vi "Conversion de Alarmas.vi"(9 "Fuente":string, 10 "Data Alarms":i16[](array[numeric])) -> (2 "Description Alarms":string[](array[string]))   [LabVIEW 2018]
doc: "Convierte el Array I16 que representa la tabla Status.Alarms a un Array String que representa la lista de alarmas del sistema."
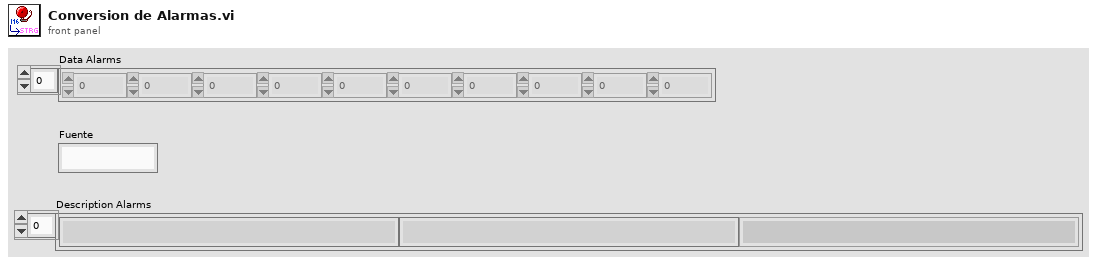
[diagram p1: front panel]
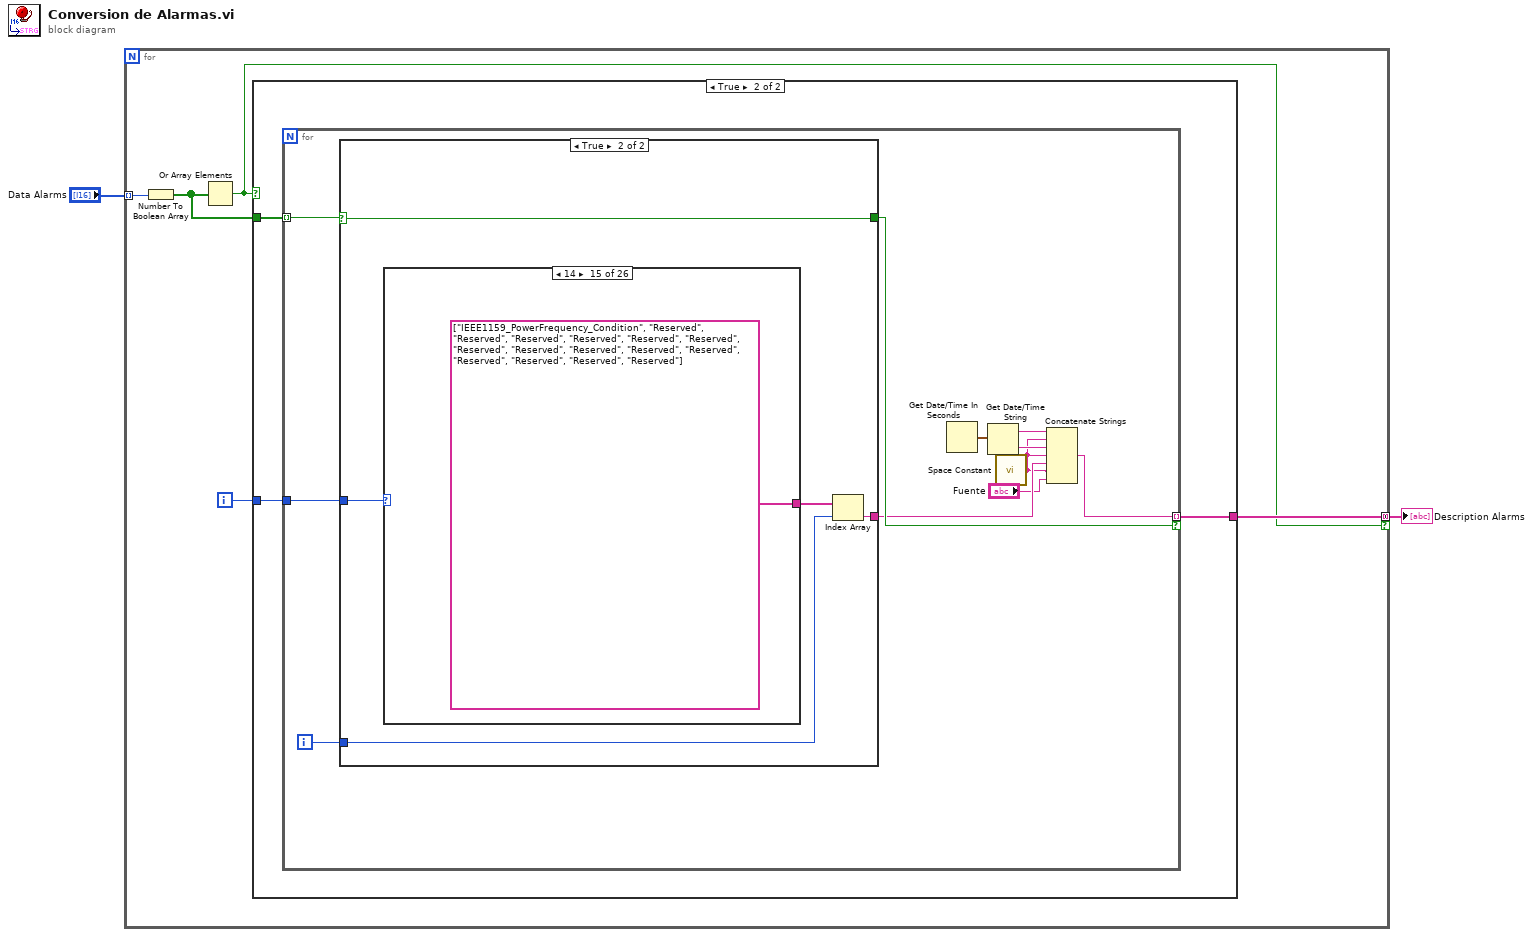
[diagram p0: block diagram]
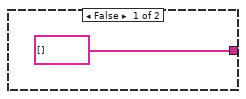
[diagram p2: hidden frame]
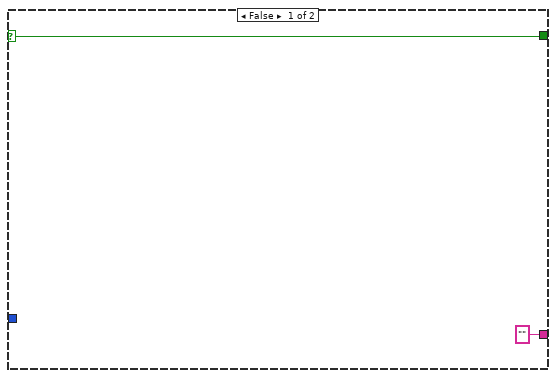
[diagram p3: hidden frame]
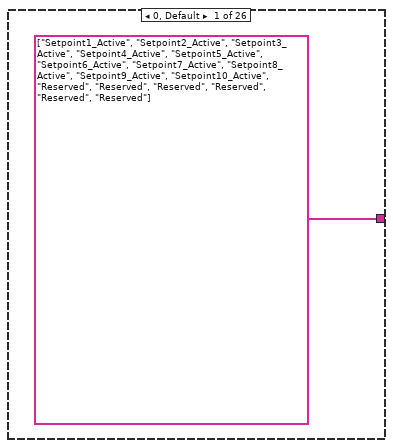
[diagram p4: hidden frame]
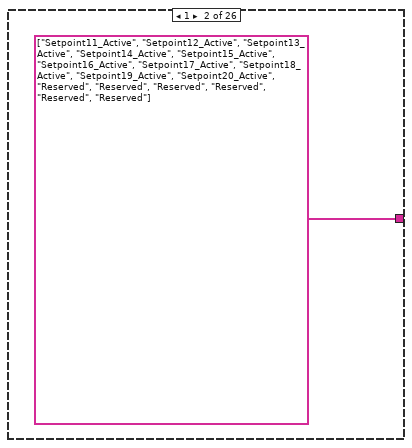
[diagram p5: hidden frame]
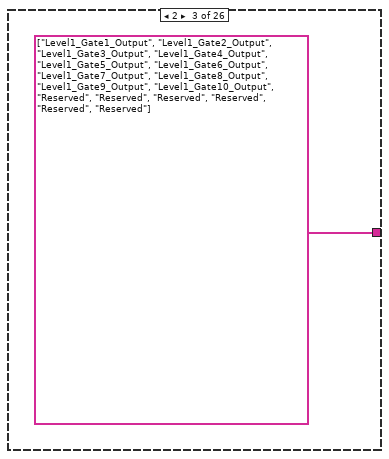
[diagram p6: hidden frame]
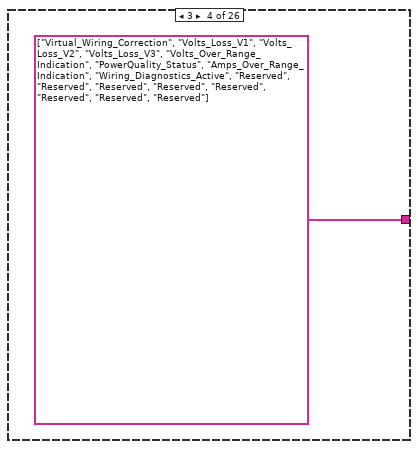
[diagram p7: hidden frame]
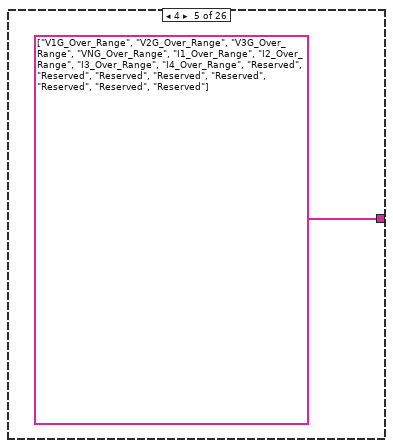
[diagram p8: hidden frame]
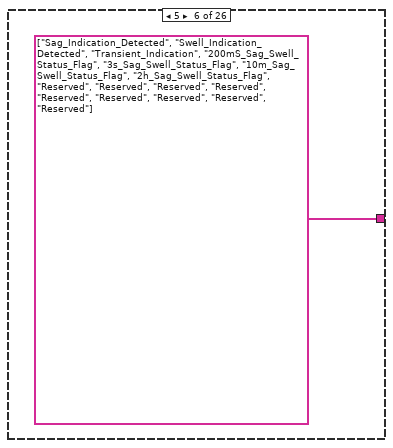
[diagram p9: hidden frame]
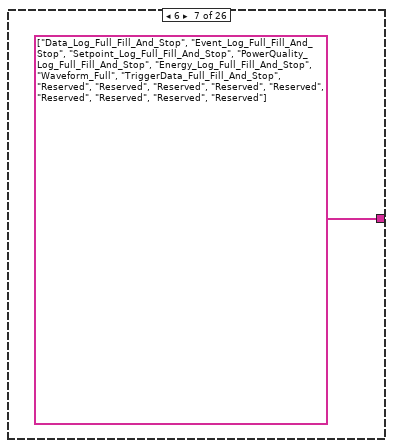
[diagram p10: hidden frame]
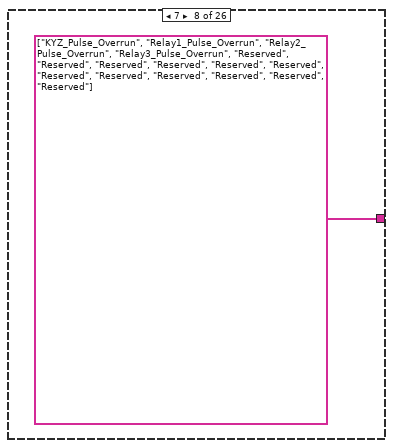
[diagram p11: hidden frame]
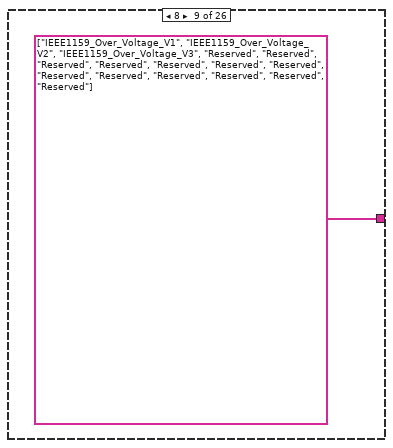
[diagram p12: hidden frame]
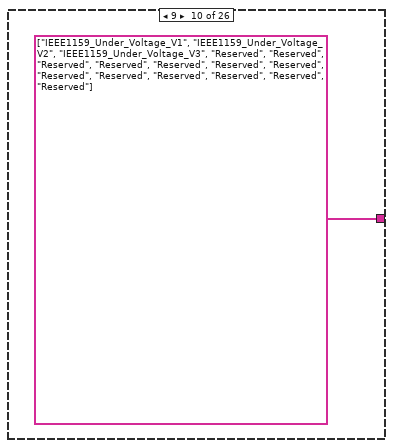
[diagram p13: hidden frame]
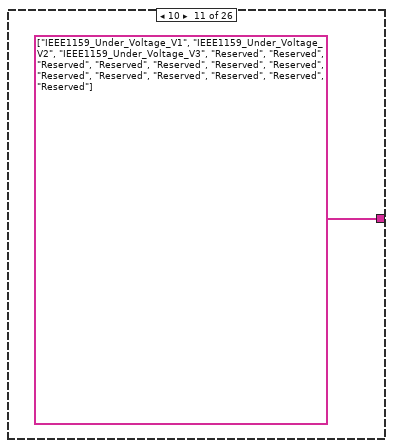
[diagram p14: hidden frame]
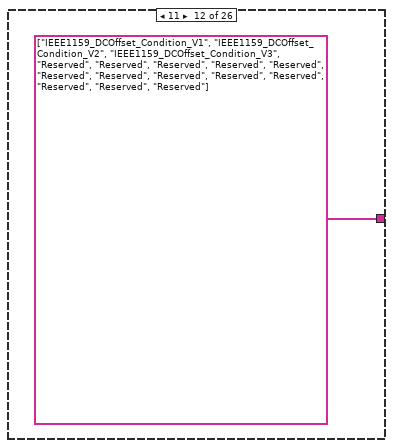
[diagram p15: hidden frame]
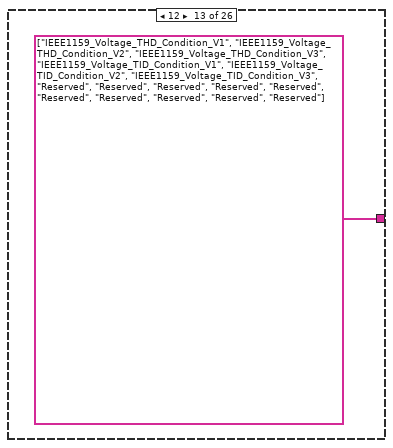
[diagram p16: hidden frame]
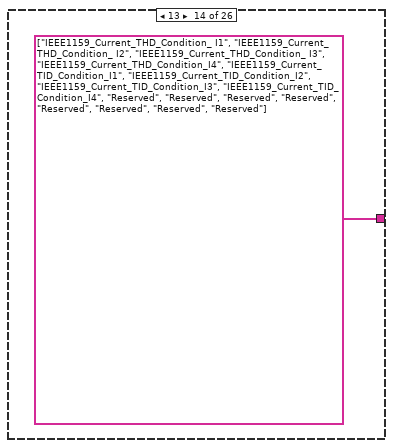
[diagram p17: hidden frame]
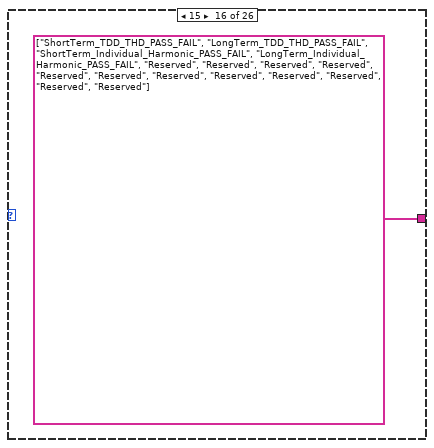
[diagram p18: hidden frame]
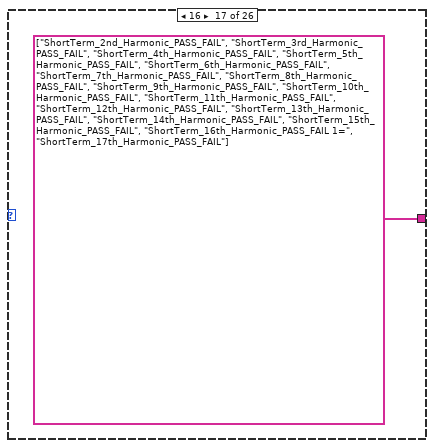
[diagram p19: hidden frame]
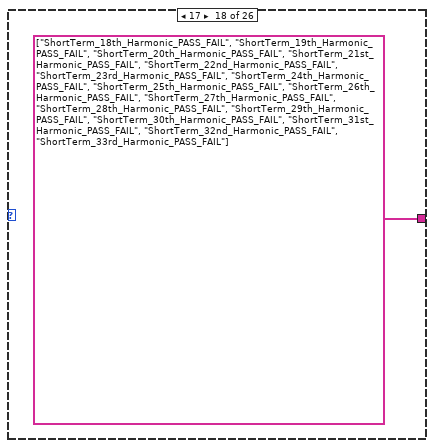
[diagram p20: hidden frame]
diagram:
  n1 = for {
    tunnel: [w5] -> w2 mode=concatenating if=w4
    tunnel: "Data Alarms" -> [w3] mode=indexing
    i -> [w7]
    n2 = Number To Boolean Array(number=w3) -> (Boolean array=w6:bool[])
    n3 = Or Array Elements(Boolean array=w6) -> (logical OR=w4:bool)
    n4 = case shown="True" w4 {
      tunnel: w7 -> [_ w10]
      tunnel: w6 -> [_ w11]
      tunnel: [string[] [] w9] -> w5
      frame False {
      }
      frame True {
        n5 = for {
          tunnel: w11 -> [w21] mode=indexing
          tunnel: w10 -> [w22]
          tunnel: [w14] -> w9 mode=indexing if=w19
          i -> [w20]
          n6 = case shown="True" w21 {
            selector: w21 -> [w23 w25]
            tunnel: w22 -> [_ w29]
            tunnel: w20 -> [_ w27]
            tunnel: ["" w26] -> w15
            tunnel: [w23 w25] -> w19
            frame False {
            }
            frame True {
              n7 = case shown="14" w29 {
                tunnel: [string[] ["Setpoint1_Active", "Setpoint2_Active", "Setpoint3_Active", "Setpoint4_Active", "Setpoint5_Active", "Setpoint6_Active", "Setpoint7_Active", "Setpoint8_Active", "Setpoint9_Active", "Setpoint10_Active", "Reserved", "Reserved", "Reserved", "Reserved", "Reserved", "Reserved"] string[] ["Setpoint11_Active", "Setpoint12_Active", "Setpoint13_Active", "Setpoint14_Active", "Setpoint15_Active", "Setpoint16_Active", "Setpoint17_Active", "Setpoint18_Active", "Setpoint19_Active", "Setpoint20_Active", "Reserved", "Reserved", "Reserved", "Reserved", "Reserved", "Reserved"] string[] ["Level1_Gate1_Output", "Level1_Gate2_Output", "Level1_Gate3_Output", "Level1_Gate4_Output", "Level1_Gate5_Output", "Level1_Gate6_Output", "Level1_Gate7_Output", "Level1_Gate8_Output", "Level1_Gate9_Output", "Level1_Gate10_Output", "Reserved", "Reserved", "Reserved", "Reserved", "Reserved", "Reserved"] string[] ["Virtual_Wiring_Correction", "Volts_Loss_V1", "Volts_Loss_V2", "Volts_Loss_V3", "Volts_Over_Range_Indication", "PowerQuality_Status", "Amps_Over_Range_Indication", "Wiring_Diagnostics_Active", "Reserved", "Reserved", "Reserved", "Reserved", "Reserved", "Reserved", "Reserved", "Reserved"] string[] ["V1G_Over_Range", "V2G_Over_Range", "V3G_Over_Range", "VNG_Over_Range", "I1_Over_Range", "I2_Over_Range", "I3_Over_Range", "I4_Over_Range", "Reserved", "Reserved", "Reserved", "Reserved", "Reserved", "Reserved", "Reserved", "Reserved"] string[] ["Sag_Indication_Detected", "Swell_Indication_Detected", "Transient_Indication", "200mS_Sag_Swell_Status_Flag", "3s_Sag_Swell_Status_Flag", "10m_Sag_Swell_Status_Flag", "2h_Sag_Swell_Status_Flag", "Reserved", "Reserved", "Reserved", "Reserved", "Reserved", "Reserved", "Reserved", "Reserved", "Reserved"] string[] ["Data_Log_Full_Fill_And_Stop", "Event_Log_Full_Fill_And_Stop", "Setpoint_Log_Full_Fill_And_Stop", "PowerQuality_Log_Full_Fill_And_Stop", "Energy_Log_Full_Fill_And_Stop", "Waveform_Full", "TriggerData_Full_Fill_And_Stop", "Reserved", "Reserved", "Reserved", "Reserved", "Reserved", "Reserved", "Reserved", "Reserved", "Reserved"] string[] ["KYZ_Pulse_Overrun", "Relay1_Pulse_Overrun", "Relay2_Pulse_Overrun", "Relay3_Pulse_Overrun", "Reserved", "Reserved", "Reserved", "Reserved", "Reserved", "Reserved", "Reserved", "Reserved", "Reserved", "Reserved", "Reserved", "Reserved"] string[] ["IEEE1159_Over_Voltage_V1", "IEEE1159_Over_Voltage_V2", "IEEE1159_Over_Voltage_V3", "Reserved", "Reserved", "Reserved", "Reserved", "Reserved", "Reserved", "Reserved", "Reserved", "Reserved", "Reserved", "Reserved", "Reserved", "Reserved"] string[] ["IEEE1159_Under_Voltage_V1", "IEEE1159_Under_Voltage_V2", "IEEE1159_Under_Voltage_V3", "Reserved", "Reserved", "Reserved", "Reserved", "Reserved", "Reserved", "Reserved", "Reserved", "Reserved", "Reserved", "Reserved", "Reserved", "Reserved"] string[] ["IEEE1159_Under_Voltage_V1", "IEEE1159_Under_Voltage_V2", "IEEE1159_Under_Voltage_V3", "Reserved", "Reserved", "Reserved", "Reserved", "Reserved", "Reserved", "Reserved", "Reserved", "Reserved", "Reserved", "Reserved", "Reserved", "Reserved"] string[] ["IEEE1159_DCOffset_Condition_V1", "IEEE1159_DCOffset_Condition_V2", "IEEE1159_DCOffset_Condition_V3", "Reserved", "Reserved", "Reserved", "Reserved", "Reserved", "Reserved", "Reserved", "Reserved", "Reserved", "Reserved", "Reserved", "Reserved", "Reserved"] string[] ["IEEE1159_Voltage_THD_Condition_V1", "IEEE1159_Voltage_THD_Condition_V2", "IEEE1159_Voltage_THD_Condition_V3", "IEEE1159_Voltage_TID_Condition_V1", "IEEE1159_Voltage_TID_Condition_V2", "IEEE1159_Voltage_TID_Condition_V3", "Reserved", "Reserved", "Reserved", "Reserved", "Reserved", "Reserved", "Reserved", "Reserved", "Reserved", "Reserved"] string[] ["IEEE1159_Current_THD_Condition_ I1", "IEEE1159_Current_THD_Condition_ I2", "IEEE1159_Current_THD_Condition_ I3", "IEEE1159_Current_THD_Condition_I4", "IEEE1159_Current_TID_Condition_I1", "IEEE1159_Current_TID_Condition_I2", "IEEE1159_Current_TID_Condition_I3", "IEEE1159_Current_TID_Condition_I4", "Reserved", "Reserved", "Reserved", "Reserved", "Reserved", "Reserved", "Reserved", "Reserved"] string[] ["IEEE1159_PowerFrequency_Condition", "Reserved", "Reserved", "Reserved", "Reserved", "Reserved", "Reserved", "Reserved", "Reserved", "Reserved", "Reserved", "Reserved", "Reserved", "Reserved", "Reserved", "Reserved"] string[] ["ShortTerm_TDD_THD_PASS_FAIL", "LongTerm_TDD_THD_PASS_FAIL", "ShortTerm_Individual_Harmonic_PASS_FAIL", "LongTerm_Individual_Harmonic_PASS_FAIL", "Reserved", "Reserved", "Reserved", "Reserved", "Reserved", "Reserved", "Reserved", "Reserved", "Reserved", "Reserved", "Reserved", "Reserved"] string[] ["ShortTerm_2nd_Harmonic_PASS_FAIL", "ShortTerm_3rd_Harmonic_PASS_FAIL", "ShortTerm_4th_Harmonic_PASS_FAIL", "ShortTerm_5th_Harmonic_PASS_FAIL", "ShortTerm_6th_Harmonic_PASS_FAIL", "ShortTerm_7th_Harmonic_PASS_FAIL", "ShortTerm_8th_Harmonic_PASS_FAIL", "ShortTerm_9th_Harmonic_PASS_FAIL", "ShortTerm_10th_Harmonic_PASS_FAIL", "ShortTerm_11th_Harmonic_PASS_FAIL", "ShortTerm_12th_Harmonic_PASS_FAIL", "ShortTerm_13th_Harmonic_PASS_FAIL", "ShortTerm_14th_Harmonic_PASS_FAIL", "ShortTerm_15th_Harmonic_PASS_FAIL", "ShortTerm_16th_Harmonic_PASS_FAIL 1=", "ShortTerm_17th_Harmonic_PASS_FAIL"] string[] ["ShortTerm_18th_Harmonic_PASS_FAIL", "ShortTerm_19th_Harmonic_PASS_FAIL", "ShortTerm_20th_Harmonic_PASS_FAIL", "ShortTerm_21st_Harmonic_PASS_FAIL", "ShortTerm_22nd_Harmonic_PASS_FAIL", "ShortTerm_23rd_Harmonic_PASS_FAIL", "ShortTerm_24th_Harmonic_PASS_FAIL", "ShortTerm_25th_Harmonic_PASS_FAIL", "ShortTerm_26th_Harmonic_PASS_FAIL", "ShortTerm_27th_Harmonic_PASS_FAIL", "ShortTerm_28th_Harmonic_PASS_FAIL", "ShortTerm_29th_Harmonic_PASS_FAIL", "ShortTerm_30th_Harmonic_PASS_FAIL", "ShortTerm_31st_Harmonic_PASS_FAIL", "ShortTerm_32nd_Harmonic_PASS_FAIL", "ShortTerm_33rd_Harmonic_PASS_FAIL"] string[] ["ShortTerm_34th_Harmonic_PASS_FAIL", "ShortTerm_35th_Harmonic_PASS_FAIL", "ShortTerm_36th_Harmonic_PASS_FAIL", "ShortTerm_37th_Harmonic_PASS_FAIL", "ShortTerm_38th_Harmonic_PASS_FAIL", "ShortTerm_39th_Harmonic_PASS_FAIL", "ShortTerm_40th_Harmonic_PASS_FAIL", "Reserved", "Reserved", "Reserved", "Reserved", "Reserved", "Reserved", "Reserved", "Reserved", "Reserved"] string[] ["LongTerm_2nd_Harmonic_PASS_FAIL", "LongTerm_3rd_Harmonic_PASS_FAIL", "LongTerm_4th_Harmonic_PASS_FAIL", "LongTerm_5th_Harmonic_PASS_FAIL", "LongTerm_6th_Harmonic_PASS_FAIL", "LongTerm_7th_Harmonic_PASS_FAIL", "LongTerm_8th_Harmonic_PASS_FAIL", "LongTerm_9th_Harmonic_PASS_FAIL", "LongTerm_10th_Harmonic_PASS_FAIL", "LongTerm_11th_Harmonic_PASS_FAIL", "LongTerm_12th_Harmonic_PASS_FAIL", "LongTerm_13th_Harmonic_PASS_FAIL", "LongTerm_14th_Harmonic_PASS_FAIL", "LongTerm_15th_Harmonic_PASS_FAIL", "LongTerm_16th_Harmonic_PASS_FAIL", "LongTerm_17th_Harmonic_PASS_FAIL"] string[] ["LongTerm_18th_Harmonic_PASS_FAIL", "LongTerm_19th_Harmonic_PASS_FAIL", "LongTerm_20th_Harmonic_PASS_FAIL", "LongTerm_21st_Harmonic_PASS_FAIL", "LongTerm_22nd_Harmonic_PASS_FAIL", "LongTerm_23rd_Harmonic_PASS_FAIL", "LongTerm_24th_Harmonic_PASS_FAIL", "LongTerm_25th_Harmonic_PASS_FAIL", "LongTerm_26th_Harmonic_PASS_FAIL", "LongTerm_27th_Harmonic_PASS_FAIL", "LongTerm_28th_Harmonic_PASS_FAIL", "LongTerm_29th_Harmonic_PASS_FAIL", "LongTerm_30th_Harmonic_PASS_FAIL", "LongTerm_31st_Harmonic_PASS_FAIL", "LongTerm_32nd_Harmonic_PASS_FAIL", "LongTerm_33rd_Harmonic_PASS_FAIL"] string[] ["LongTerm_34th_Harmonic_PASS_FAIL", "LongTerm_35th_Harmonic_PASS_FAIL", "LongTerm_36th_Harmonic_PASS_FAIL", "LongTerm_37th_Harmonic_PASS_FAIL", "LongTerm_38th_Harmonic_PASS_FAIL", "LongTerm_39th_Harmonic_PASS_FAIL", "LongTerm_40th_Harmonic_PASS_FAIL", "Reserved", "Reserved", "Reserved", "Reserved", "Reserved", "Reserved", "Reserved", "Reserved", "Reserved"] string[] ["IEEE1159_Voltage_Fluctuation_V1", "IEEE1159_Voltage_Fluctuation_V2", "IEEE1159_Voltage_Fluctuation_V3", "Reserved", "Reserved", "Reserved", "Reserved", "Reserved", "Reserved", "Reserved", "Reserved", "Reserved", "Reserved", "Reserved", "Reserved", "Reserved"] string[] ["EN61000_4_30_Mains_Signaling_V1", "EN61000_4_30_Mains_Signaling_V2", "EN61000_4_30_Mains_Signaling_V3", "Reserved", "Reserved", "Reserved", "Reserved", "Reserved", "Reserved", "Reserved", "Reserved", "Reserved", "Reserved", "Reserved", "Reserved", "Reserved"] string[] ["EN61000_4_30_Under_Deviation_V1", "EN61000_4_30_Under_Deviation_V2", "EN61000_4_30_Under_Deviation_V3", "Reserved", "Reserved", "Reserved", "Reserved", "Reserved", "Reserved", "Reserved", "Reserved", "Reserved", "Reserved", "Reserved", "Reserved", "Reserved"] string[] ["EN61000_4_30_Over_Deviation_V1", "EN61000_4_30_Over_Deviation_V2", "EN61000_4_30_Over_Deviation_V3", "Reserved", "Reserved", "Reserved", "Reserved", "Reserved", "Reserved", "Reserved", "Reserved", "Reserved", "Reserved", "Reserved", "Reserved", "Reserved"]] -> w28
                frame 0, Default {
                }
                frame 1 {
                }
                frame 2 {
                }
                frame 3 {
                }
                frame 4 {
                }
                frame 5 {
                }
                frame 6 {
                }
                frame 7 {
                }
                frame 8 {
                }
                frame 9 {
                }
                frame 10 {
                }
                frame 11 {
                }
                frame 12 {
                }
                frame 13 {
                }
                frame 14 {
                }
                frame 15 {
                }
                frame 16 {
                }
                frame 17 {
                }
                frame 18 {
                }
                frame 19 {
                }
                frame 20 {
                }
                frame 21 {
                }
                frame 22 {
                }
                frame 23 {
                }
                frame 24 {
                }
                frame 25 {
                }
              }
              n8 = Index Array(array=w28, index=w27) -> (element=w26:string)
            }
          }
          n9 = Get Date/Time In Seconds() -> (seconds since 1Jan1904=w17:timestamp)
          n10 = Get Date/Time String(seconds (now)=w17) -> (date string=w16:string, time string=w18:string)  [unwired: 2 in]
          n11 = call <vilib>:"Space Constant.vi"() -> ("String"=w13:string)
          n12 = Concatenate Strings(w16, w13, w18, w13, w15, w13, "Fuente") -> (w14:string)
        }
      }
    }
  }
  "Description Alarms" <- w2
